vi "Remove Controls from Selection Target.vi"() -> ()   [LabVIEW 2018, in "Tests.lvlib" / "Toolkit.lvlib" / "Unit.lvlib"]
uses:
  Unit.lvlib
panel:
  out "Any?":bool
  in  "Input":bool[](array[boolean])
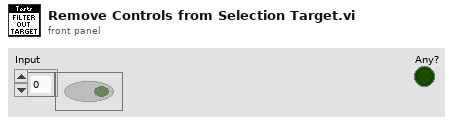
[diagram p1: front panel]
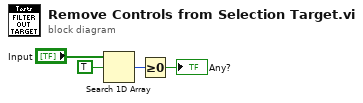
[diagram p0: block diagram]
diagram:
  n1 = Search 1D Array(1D array="Input", element=TRUE) -> (index of element=w3:i32)  [unwired: 1 in]
  n2 = Greater Or Equal To 0?(x=w3) -> (x >= 0?=→"Any?":bool)
